vi "Write Cancel ref.vi"(10 "Cancel build ref":refnum<vi>, 11 "BuildManager in":refnum<class "BuildManager.lvclass">) -> (3 "BuildManager out":refnum<class "BuildManager.lvclass">)   [LabVIEW 2019, in "SolutionBuilder.lvlib" / "BuildManager.lvclass"]
uses:
  BuildManager.lvclass
  BuildManager.lvclass/BuildManager.ctl
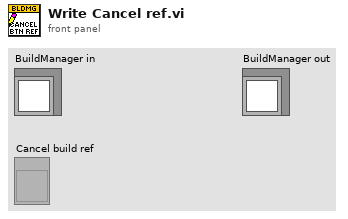
[diagram p1: front panel]
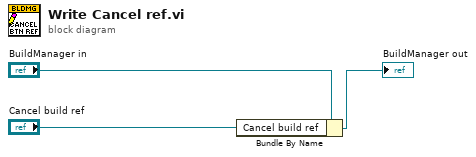
[diagram p0: block diagram]
diagram:
  n1 = Bundle By Name(cluster="BuildManager in", "Cancel build ref"="Cancel build ref") -> (→"BuildManager out":refnum<class "BuildManager.lvclass">)
